vi "Intrinsic Sensors.vi"(8 "error in (no error)":errorcluster, 11 "output cluster":T1) -> (0 "error out":errorcluster)   [LabVIEW 2016]
uses:
  Queue Cluster TD.ctl
  Queue Attributes TD.ctl
  Queue Enum TD.ctl
  Intrinsic Data TD.ctl
  <vilib>/addons/zeromq/socket_type.ctl
  <vilib>/addons/zeromq/socket_options.ctl
  <vilib>/addons/zeromq/zeromq.lvlib
  <vilib>/addons/zeromq/zmq_context.lvclass
  <vilib>/addons/zeromq/zmq_socket.lvclass
panel:
  out "Intrinsic Sensors":cluster{dbl, dbl, dbl}(graph)
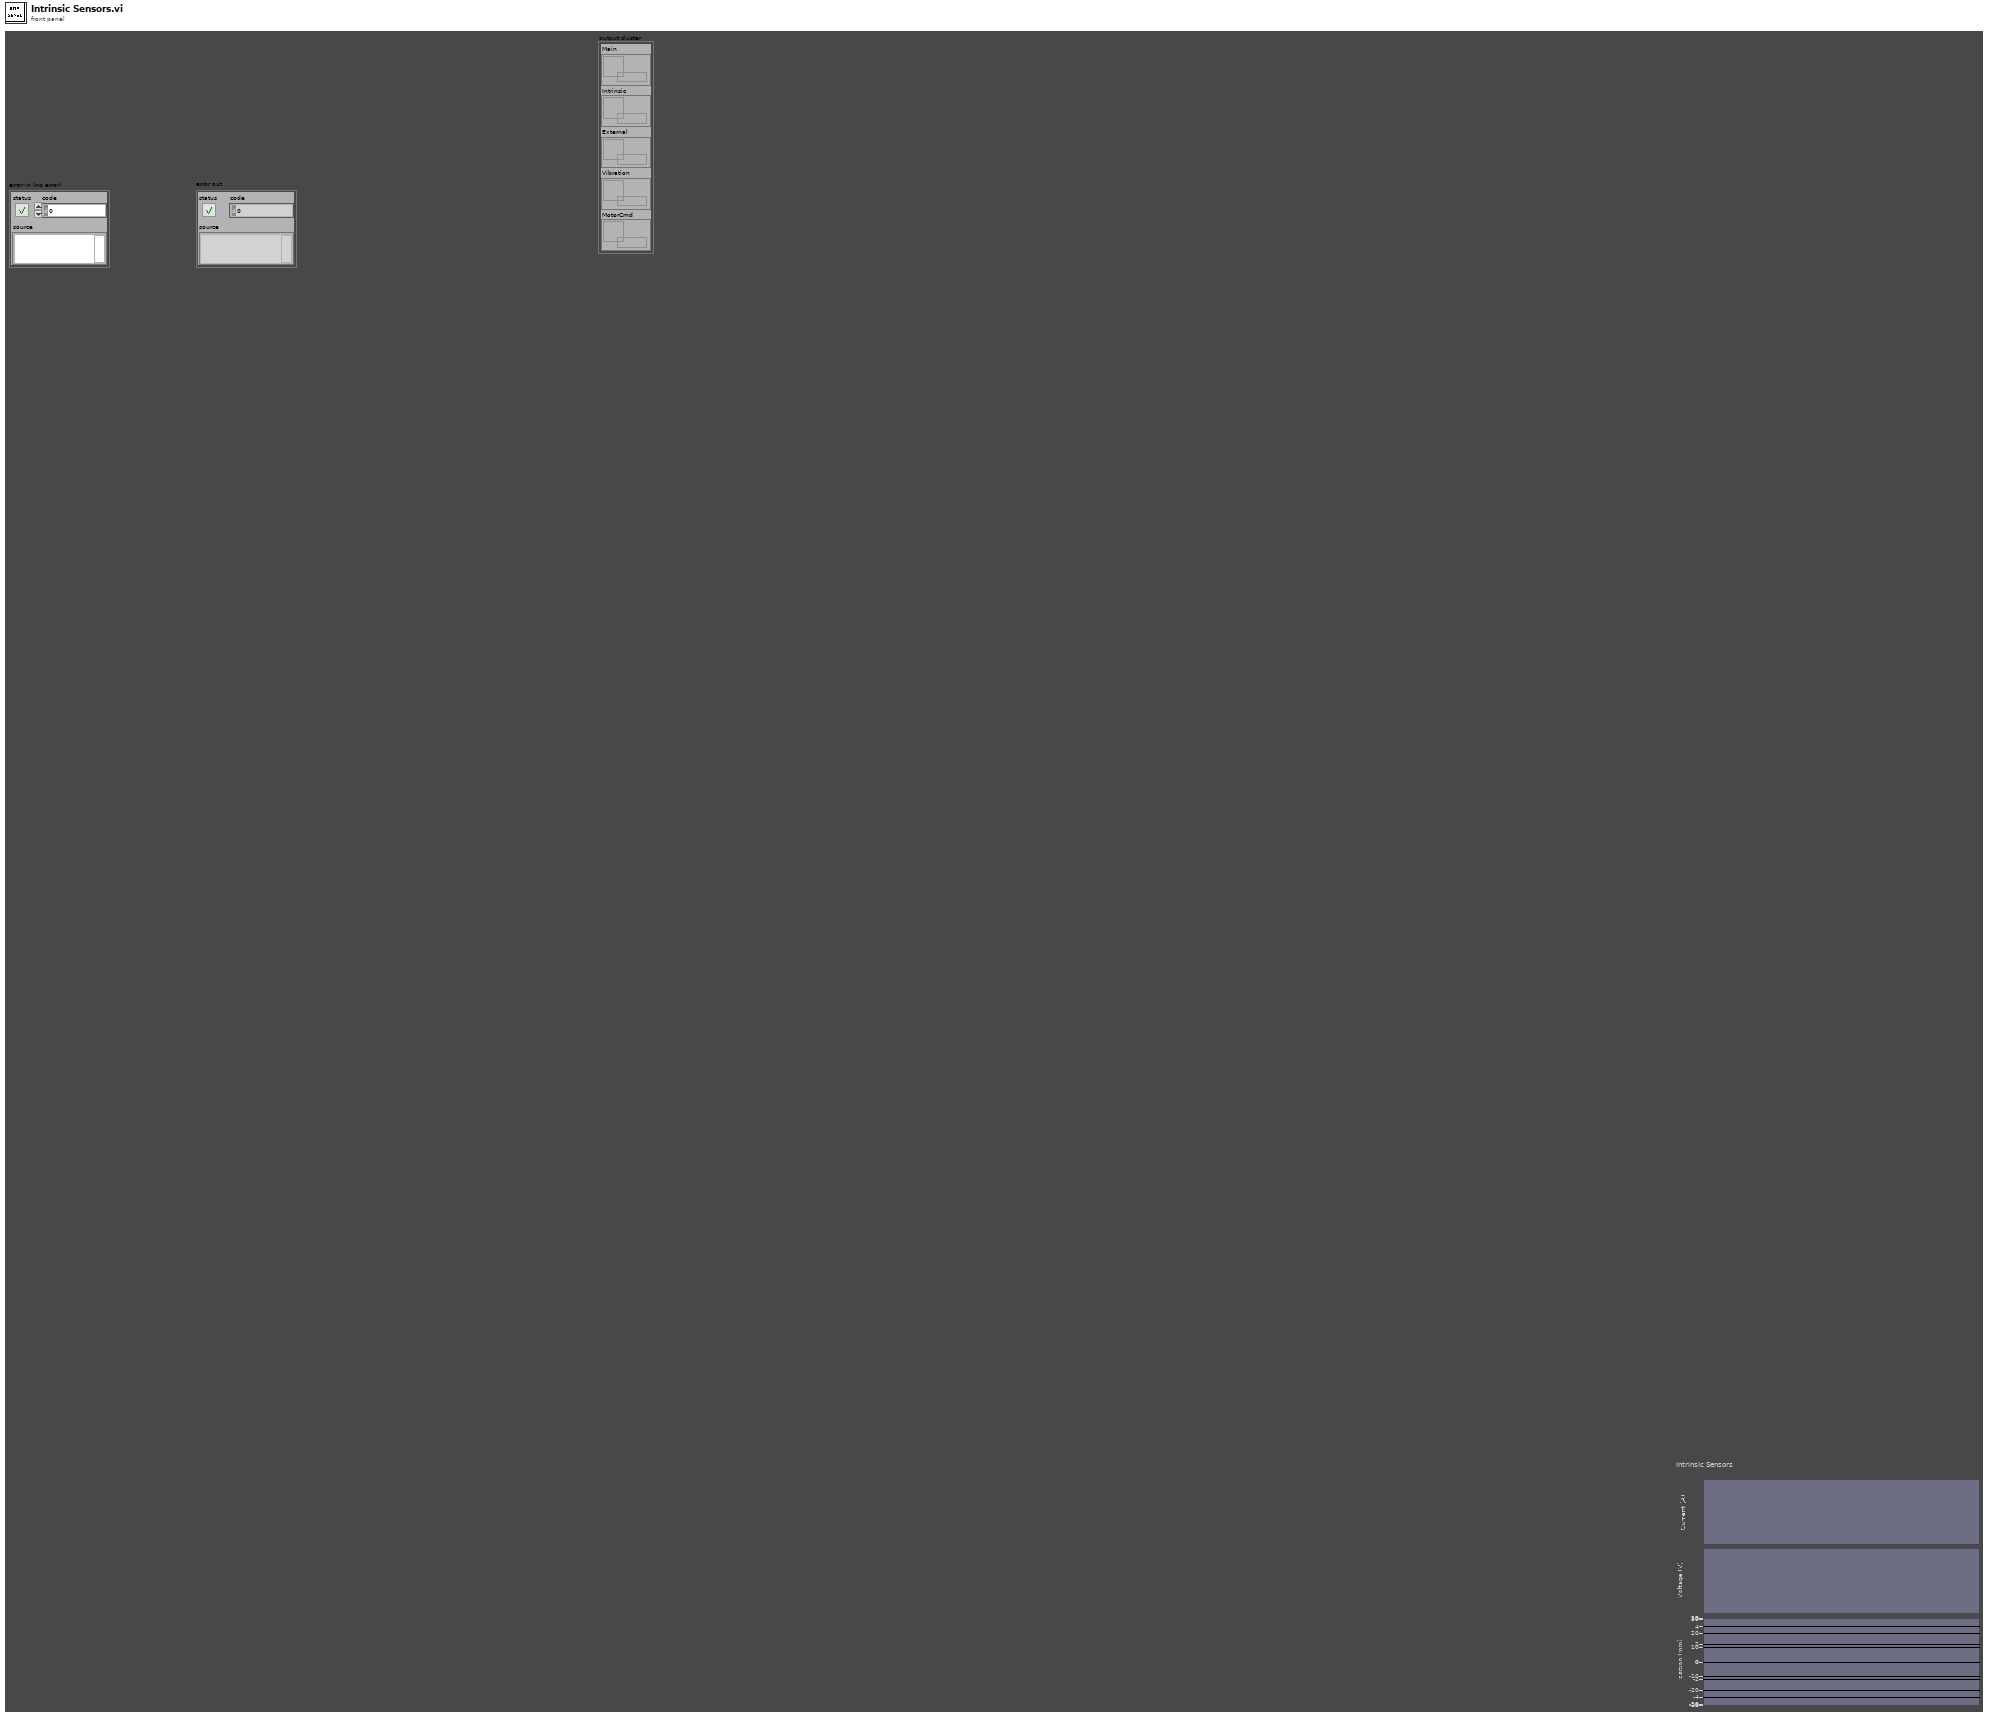
[diagram p1: front panel]
types:
  T1 = typedef "Queue Cluster TD.ctl" = cluster{"Main":refnum<queue>, "Intrinsic":refnum<queue>, "External":refnum<queue>, "Vibration":refnum<queue>, "MotorCmd":refnum<queue>}
  T2 = typedef "Intrinsic data TD.ctl" = cluster{"Current TS":string, "Current Data":string, "Voltage TS":string, "Voltage Data":string, "Position TS":string, "Position Data":string, "Connected?":bool, "Log File Refnum":refnum<file>, "Logging?":bool, "Plot?":bool, "LV_C_TS":dbl, "LV_P_TS":dbl, "LV_V_TS":dbl}
  T3 = typedef "Queue Attributes TD.ctl" = cluster{"State":T4, "String":string, "Boolean":bool, "Double":dbl, "U16":u16}
  T4 = typedef "Queue Enum TD.ctl" = enum16{"Stop", "Start", "Update D_HW", "Initialize", "Exit", "Read", "Write", "Plot", "Log", "Stop Log", "Start Log", "Wait"}
  T5 = typedef "zeromq.lvlib/socket_options.ctl" = enum8{"NONE", "ZMQ_HWM", "<2>", "ZMQ_SWAP", "ZMQ_AFFINITY", "ZMQ_IDENTITY", "ZMQ_SUBSCRIBE", "ZMQ_UNSUBSCRIBE", "ZMQ_RATE", "ZMQ_RECOVERY_IVL", "ZMQ_MCAST_LOOP", "ZMQ_SNDBUF", "ZMQ_RCVBUF", "ZMQ_RCVMORE", "ZMQ_FD", "ZMQ_EVENTS", "ZMQ_TYPE", "ZMQ_LINGER", "ZMQ_RECONNECT_IVL", "ZMQ_BACKLOG", "ZMQ_RECOVERY_IVL_MSEC", "ZMQ_RECONNECT_IVL_MAX", "ZMQ_MAXMSGSIZE", "ZMQ_SNDHWM", "ZMQ_RCVHWM", "ZMQ_MULTICAST_HOPS", "<26>", "ZMQ_RCVTIMEO", "ZMQ_SNDTIMEO", "<29>", "<30>", "ZMQ_IPV4ONLY", "ZMQ_LAST_ENDPOINT", "ZMQ_ROUTER_MANDATORY", "ZMQ_TCP_KEEPALIVE", "ZMQ_TCP_KEEPALIVE_CNT", "ZMQ_TCP_KEEPALIVE_IDLE", "ZMQ_TCP_KEEPALIVE_INTVL", "ZMQ_TCP_ACCEPT_FILTER", "ZMQ_DELAY_ATTACH_ON_CONNECT", "ZMQ_XPUB_VERBOSE"}
  T6 = typedef "zeromq.lvlib/socket_type.ctl" = enum8{"ZMQ_PAIR", "ZMQ_PUB", "ZMQ_SUB", "ZMQ_REQ", "ZMQ_REP", "ZMQ_DEALER", "ZMQ_ROUTER", "ZMQ_PULL", "ZMQ_PUSH", "ZMQ_XPUB", "ZMQ_XSUB"}
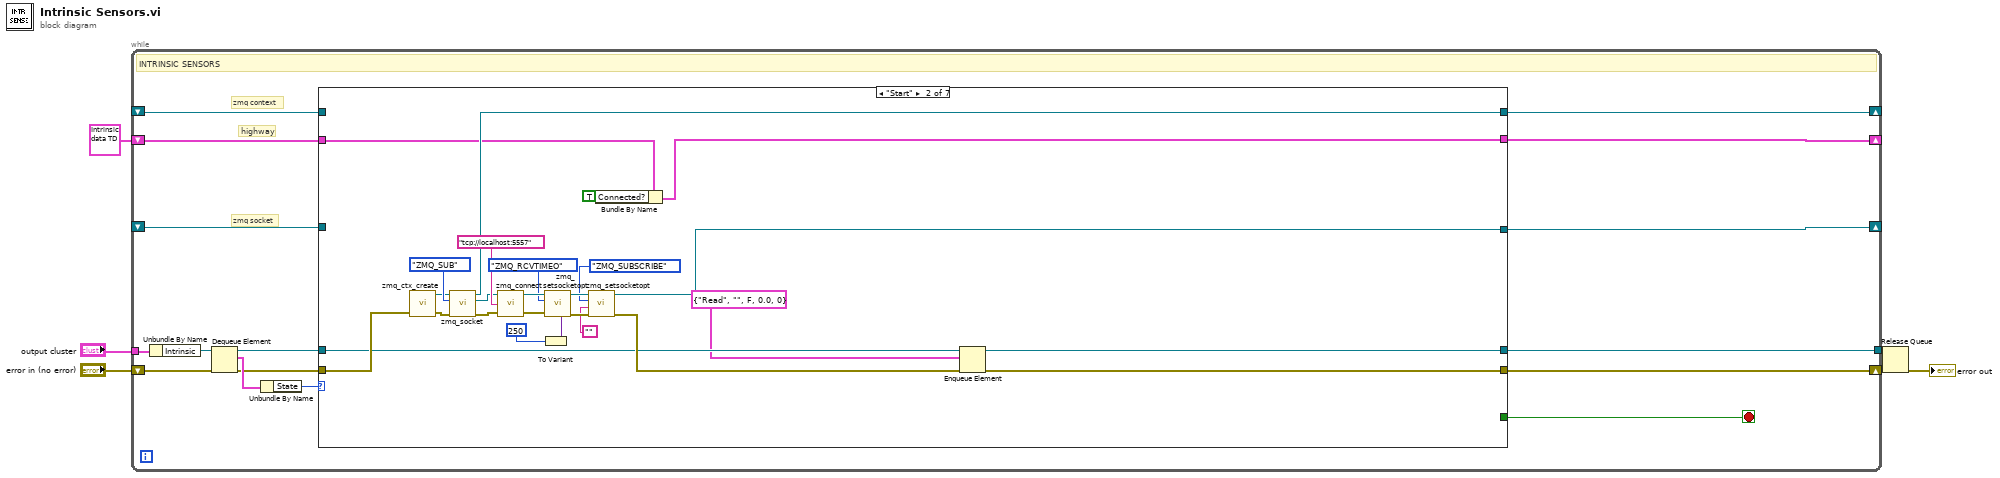
[diagram p0: block diagram]
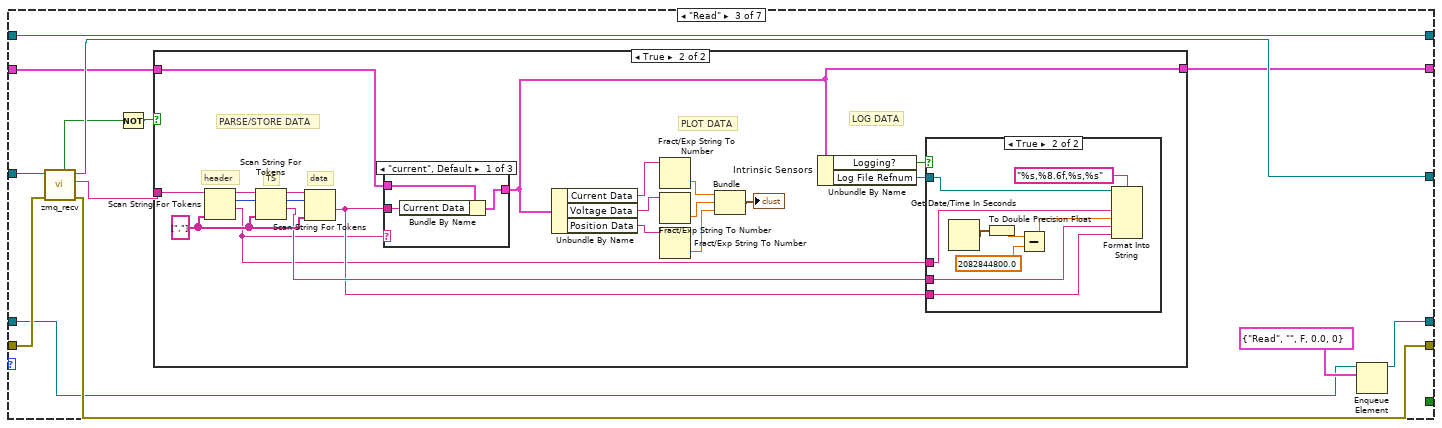
[diagram p3: hidden frame]
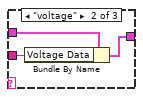
[diagram p6: hidden frame]
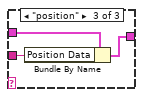
[diagram p7: hidden frame]
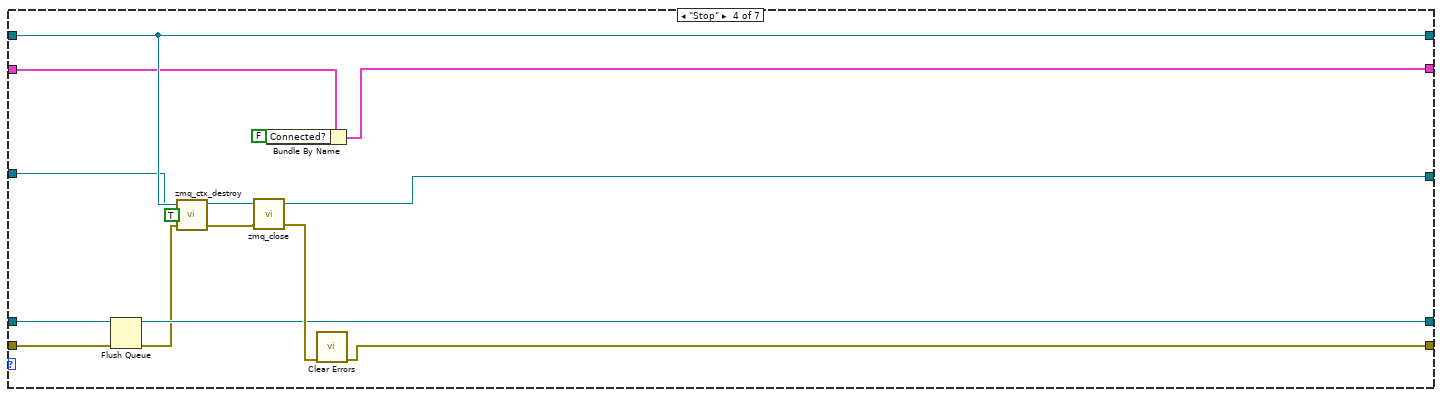
[diagram p8: hidden frame]
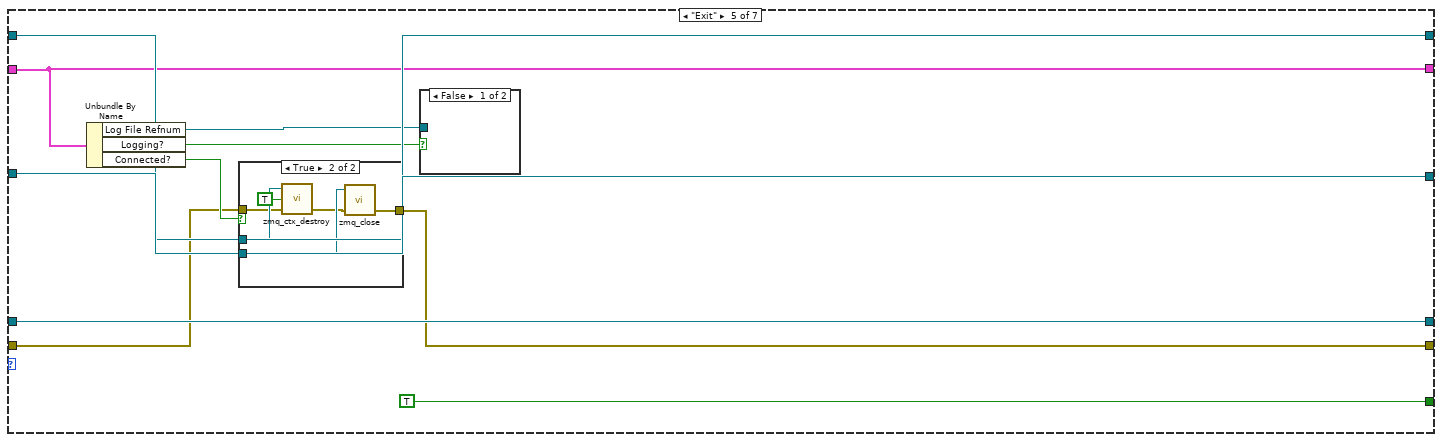
[diagram p9: hidden frame]
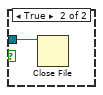
[diagram p10: hidden frame]
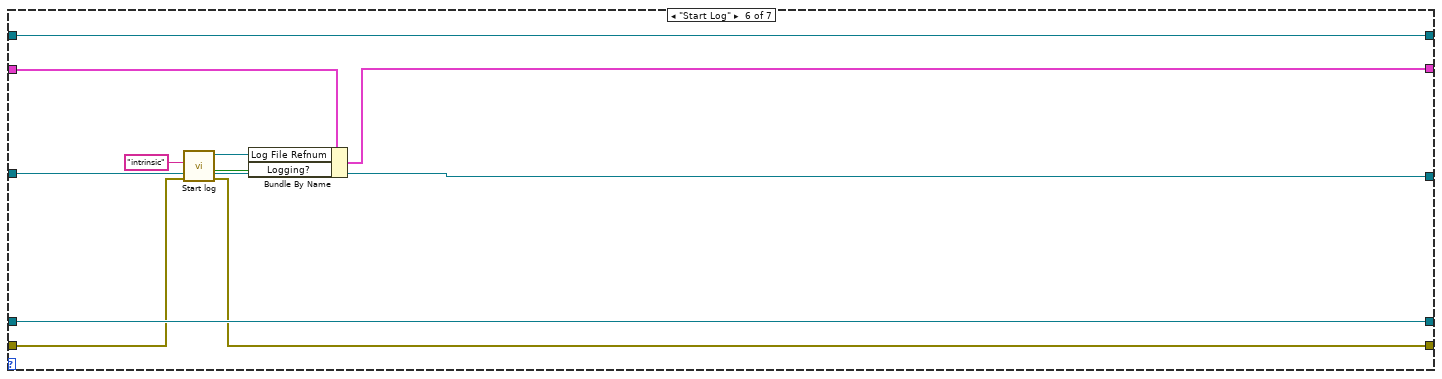
[diagram p12: hidden frame]
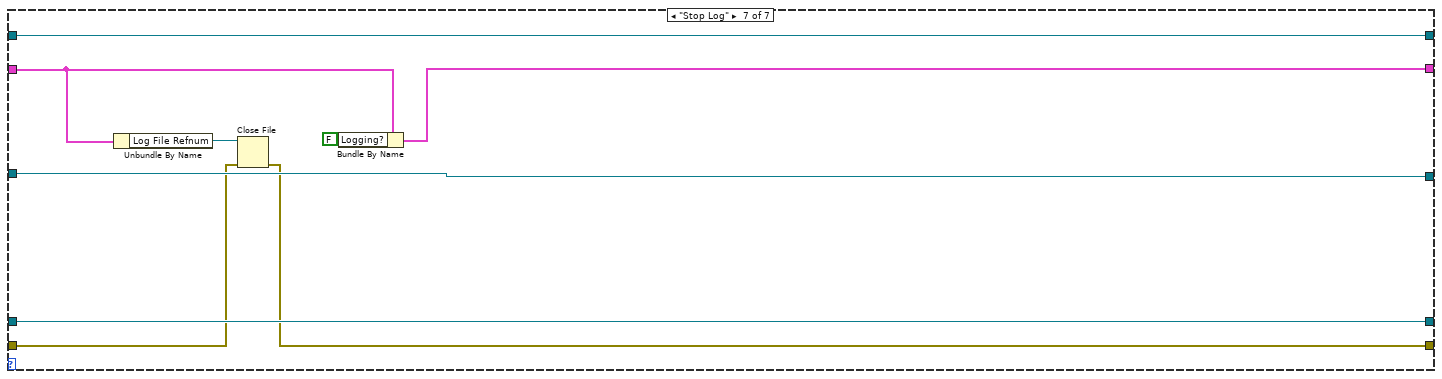
[diagram p13: hidden frame]
diagram:
  n1 = while {
    tunnel: "output cluster" -> [w22]
    tunnel: [w16] -> w5
    shift-right: [w15] -> w6
    shift-left: "error in (no error)" -> [w20]
    shift-right: [w12] -> _
    shift-left: _ -> [w11]
    shift-right: [w10] -> _
    shift-left: _ -> [w9]
    shift-right: [w7] -> _
    shift-left: T2 {"Current TS"="", "Current Data"="", "Voltage TS"="", "Voltage Data"="", "Position TS"="", "Position Data"="", "Connected?"=FALSE, "Log File Refnum"=refnum, "Logging?"=FALSE, "Plot?"=FALSE, "LV_C_TS"=0.0, "LV_P_TS"=0.0, "LV_V_TS"=0.0} ("Intrinsic Data Cluster TD") -> [w8]
    stop <- w13 stop-if-true
    # "highway"
    # "zmq socket"
    # "zmq context"
    # "INTRINSIC SENSORS"
    n2 = Unbundle By Name(w22) -> ("Intrinsic"=w21:refnum<queue>)
    n3 = Dequeue Element(queue=w21, error in (no error)=w20) -> (queue out=w17:refnum<queue>, element=w19:T3, error out=w18:errorcluster)  [unwired: 1 in, 1 out]
    n4 = Unbundle By Name(w19) -> ("State"=w14:T4)
    n5 = case shown="\"Start\"" w14 {
      tunnel: w18 -> [w26 w53 w65 w110 w120 w143 w152]
      tunnel: w17 -> [w27 w37 w58 w112 w128 w146 w155]
      tunnel: [w27 w36 w57 w111 w128 w146 w155] -> w16
      tunnel: [w26 w38 w60 w114 w119 w142 w151] -> w15
      tunnel: [_ _ _ _ TRUE _ _] -> w13
      tunnel: [w24 w34 w63 w117 w126 w145 w154] -> w12
      tunnel: w11 -> [w24 _ w64 w117 w126 w145 w154]
      tunnel: [w25 w33 w66 w118 w125 w144 w153] -> w10
      tunnel: w9 -> [w25 _ w66 w118 w125 w144 w153]
      tunnel: w8 -> [w23 w32 w62 w108 w122 w140 w148]
      tunnel: [w23 w31 w61 w107 w122 w139 w147] -> w7
      frame "Initialize", Default {
      }
      frame "Start" {
        n6 = call <vilib>:"zmq_ctx_create.vi"("error in"=w53) -> ("error out"=w45:errorcluster, "context out"=w44:refnum<class "zmq_context.lvclass">)  [unwired: 3 in]
        n7 = call <vilib>:"zmq_socket.vi"("error in"=w45, "socket type"=socket_type."ZMQ_SUB", "context in"=w44) -> ("error out"=w48:errorcluster, "socket out"=w47:refnum<class "zmq_socket.lvclass">, "context out"=w33:refnum<class "zmq_context.lvclass">)  [unwired: 2 in]
        n8 = call <vilib>:"zmq_connect.vi"("error in"=w48, "endpoint"="tcp://localhost:5557", "socket in"=w47) -> ("error out"=w52:errorcluster, "socket out"=w51:refnum<class "zmq_socket.lvclass">)  [unwired: 1 in]
        n9 = To Variant(anything=250) -> (Variant=w28:variant)
        n10 = call <vilib>:"zmq_setsocketopt.vi"("error in"=w52, "value"=w28, "option"=socket_options."ZMQ_RCVTIMEO", "socket in"=w51) -> ("error out"=w42:errorcluster, "socket out"=w43:refnum<class "zmq_socket.lvclass">)  [unwired: 2 in]
        n11 = call <vilib>:"zmq_setsocketopt.vi"("error in"=w42, "value"="", "option"=socket_options."ZMQ_SUBSCRIBE", "socket in"=w43) -> ("error out"=w39:errorcluster, "socket out"=w34:refnum<class "zmq_socket.lvclass">)  [unwired: 2 in]
        n12 = Bundle By Name(cluster=w32, "Connected?"=TRUE) -> (w31:T2)
        n13 = Enqueue Element(queue=w37, element=T3 {"State"=enum."Read", "String"="", "Boolean"=FALSE, "Double"=0.0, "U16"=0}, error in (no error)=w39) -> (queue out=w36:refnum<queue>, error out=w38:errorcluster)  [unwired: 1 in, 1 out]
      }
      frame "Read" {
        n14 = call <vilib>:"zmq_recv.vi"("error in"=w65, "socket in"=w64) -> ("error out"=w60:errorcluster, "data"=w56:string, "socket out"=w63:refnum<class "zmq_socket.lvclass">, "timeout?"=w54:bool)  [unwired: 3 in, 1 out]
        n15 = Not(x=w54) -> (.not. x?=w55:bool)
        n16 = case shown="True" w55 {
          tunnel: w62 -> [w67 w75]
          tunnel: w56 -> [_ w70]
          tunnel: [w67 w68] -> w61
          frame False {
          }
          frame True {
            w87 = string[] [","]
            # "LOG DATA"
            # "PLOT DATA"
            # "PARSE/STORE DATA"
            # "data"
            # "TS"
            # "header"
            n17 = Scan String For Tokens(6:w87, 9:w70) -> (1:w76:string, 2:w85:i32, 3:w86:string)  [unwired: 4 in, 1 out]
            n18 = Scan String For Tokens(6:w87, 8:w85, 9:w86) -> (1:w83:string, 2:w69:i32, 3:w84:string)  [unwired: 3 in, 1 out]
            n19 = Scan String For Tokens(6:w87, 8:w69, 9:w84) -> (1:w82:string)  [unwired: 3 in, 3 out]
            n20 = case shown="\"current\", Default" w76 {
              tunnel: w82 -> [w99 w102 w105]
              tunnel: [w98 w101 w104] -> w68
              tunnel: w75 -> [w97 w100 w103]
              frame "current", Default {
                n21 = Bundle By Name(cluster=w97, "Current Data"=w99) -> (w98:T2)
              }
              frame "voltage" {
                n22 = Bundle By Name(cluster=w100, "Voltage Data"=w102) -> (w101:T2)
              }
              frame "position" {
                n23 = Bundle By Name(cluster=w103, "Position Data"=w105) -> (w104:T2)
              }
            }
            n24 = Unbundle By Name(w68) -> ("Current Data"=w72:string, "Voltage Data"=w74:string, "Position Data"=w73:string)
            n25 = Fract/Exp String To Number(string=w72) -> (number=w81:dbl)  [unwired: 3 in, 1 out]
            n26 = Fract/Exp String To Number(string=w74) -> (number=w80:dbl)  [unwired: 3 in, 1 out]
            n27 = Fract/Exp String To Number(string=w73) -> (number=w79:dbl)  [unwired: 3 in, 1 out]
            n28 = Bundle(w81, w80, w79) -> (→"Intrinsic Sensors":cluster{dbl, dbl, dbl})  [unwired: 1 in]
            n29 = Unbundle By Name(w68) -> ("Logging?"=w71:bool, "Log File Refnum"=w77:refnum<file>)
            n30 = case shown="True" w71 {
              tunnel: w76 -> [_ w92]
              tunnel: w83 -> [_ w90]
              tunnel: w82 -> [_ w89]
              tunnel: w77 -> [_ w88]
              frame False {
              }
              frame True {
                n31 = Get Date/Time In Seconds() -> (seconds since 1Jan1904=w95:timestamp)
                n32 = To Double Precision Float(number=w95) -> (double precision float=w94:dbl)
                n33 = Subtract(x=w94, y=2082844800.0 ("Epoch Delta (s)")) -> (x-y=w91:dbl)
                n34 = Format Into String(format string="%s,%8.6f,%s,%s", initial string=w88, w92, w91, w90, w89) -> ()  [unwired: 1 in, 2 out]
              }
            }
          }
        }
        n35 = Enqueue Element(queue=w58, element=T3 {"State"=enum."Read", "String"="", "Boolean"=FALSE, "Double"=0.0, "U16"=0}) -> (queue out=w57:refnum<queue>)  [unwired: 2 in, 2 out]
      }
      frame "Stop" {
        n36 = Flush Queue(queue=w112, error in (no error)=w110) -> (queue out=w111:refnum<queue>, error out=w109:errorcluster)  [unwired: 1 out]
        n37 = call <vilib>:"zmq_ctx_destroy.vi"("error in"=w109, "reap? (F)"=TRUE, "context in"=w118) -> ("error out"=w116:errorcluster)  [unwired: 2 in]
        n38 = call <vilib>:"zmq_close.vi"("error in"=w116, "socket"=w117) -> ("error out"=w115:errorcluster)  [unwired: 3 in]
        n39 = Bundle By Name(cluster=w108, "Connected?"=FALSE) -> (w107:T2)
        n40 = call <vilib>:"Clear Errors.vi"("error in (no error)"=w115) -> ("error out"=w114:errorcluster)  [unwired: 5 in, 1 out]
      }
      frame "Exit" {
        n41 = Unbundle By Name(w122) -> ("Log File Refnum"=w121:refnum<file>, "Logging?"=w123:bool, "Connected?"=w124:bool)
        n42 = case shown="True" w124 {
          tunnel: w126 -> [_ w136]
          tunnel: w125 -> [_ w135]
          tunnel: w120 -> [w130 w134]
          tunnel: [w130 w132] -> w119
          frame False {
          }
          frame True {
            n43 = call <vilib>:"zmq_ctx_destroy.vi"("error in"=w134, "reap? (F)"=TRUE, "context in"=w135) -> ("error out"=w133:errorcluster)  [unwired: 2 in]
            n44 = call <vilib>:"zmq_close.vi"("error in"=w133, "socket"=w136) -> ("error out"=w132:errorcluster)  [unwired: 3 in]
          }
        }
        n45 = case shown="False" w123 {
          tunnel: w121 -> [_ w129]
          frame False {
          }
          frame True {
            n46 = Close File(refnum=w129) -> ()  [unwired: 1 in, 2 out]
          }
        }
      }
      frame "Start Log" {
        n47 = call "Start log.vi"("error in (no error)"=w143, "Filename root"="intrinsic" ("Data type")) -> ("error out"=w142:errorcluster, "Logging"=w137:bool, "Byte Stream File out"=w138:refnum<file>)  [unwired: 7 in]
        n48 = Bundle By Name(cluster=w140, "Log File Refnum"=w138, "Logging?"=w137) -> (w139:T2)
      }
      frame "Stop Log" {
        n49 = Unbundle By Name(w148) -> ("Log File Refnum"=w150:refnum<file>)
        n50 = Close File(refnum=w150, error in=w152) -> (error out=w151:errorcluster)  [unwired: 1 out]
        n51 = Bundle By Name(cluster=w148, "Logging?"=FALSE) -> (w147:T2)
      }
    }
  }
  n52 = Release Queue(queue=w5, error in (no error)=w6) -> (error out=→"error out":errorcluster)  [unwired: 1 in, 2 out]
